vi "Autocomplete Demo.vi"() -> ()   [LabVIEW 2012]
doc: "This example includes a string XControl that probes the user input and checks it against a dynamic set of keywords. If what you type matches a keyword, the XControl autocompletes the word and selects the remaining portion of the word. This is also known as intellisense. At that point the you can tab to accept the autocompletion or keep typing to overwrite the completed portion.\n\nTo view the example:\n1) Run the VI.\n2) Type words in the <b>Intellisense Xcontrol</b> text box.\n\nYou can turn the Autocomplete function on or off as well as add new keywords to the Xcontrol."
uses:
  xcontrol/Intellisense Xcontrol.xctl
  xcontrol/Properties/Delimiter/Delimiter Enum.ctl
panel:
  in  "Keyword Dialog":bool
  in  "Delimiter":T1=enum."Space"
  in  "On/Off":bool=TRUE
  in  "Keyword Array":string[](array[string])
  in  "stop":bool
  out "Output Value":string
  in  "Intellisense Xcontrol":string(xcontrol)
  # "Select Help»Show Context Help and move the cursor \nover the VI icon to display help for this VI."
  # "Type text into the string control. If autocomplete is on and the text matches\na keyword, then the Xcontrol will autocomplete the keyword. To accept the\nautocompletion and add a delimiter, press tab. Otherwise, keep tying."
  # "Turn Autocomplete\non or off"
  # "Change the delimiter that\nseparates keywords"
  # "Add new keywords or\nchange the existing ones\nthat the Xcontrol searches\nfor by entering them into\nthe array of keywords."
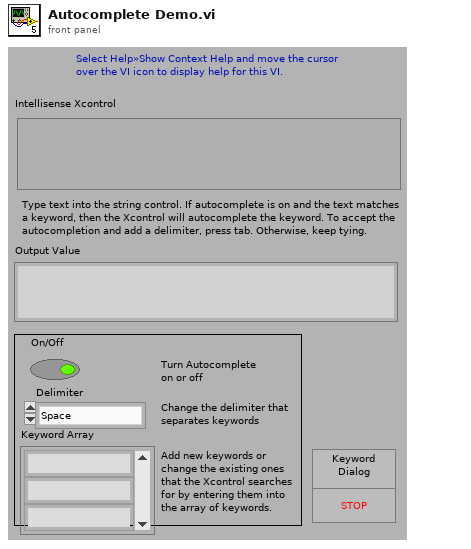
[diagram p1: front panel]
types:
  T1 = typedef "Intellisense Xcontrol.xctl/Delimiter Enum.ctl" = enum16{"None", "Space", "Dash \"-\"", "Slash \"/\"", "Backslash \"\\\"", "Colon", "Period", "Comma", "Line Feed"}
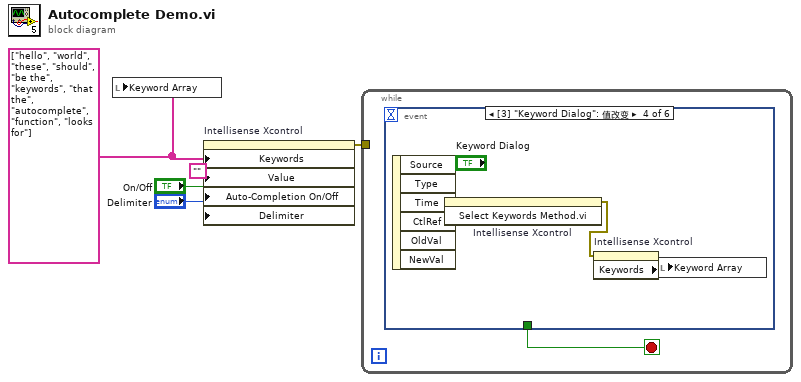
[diagram p0: block diagram]
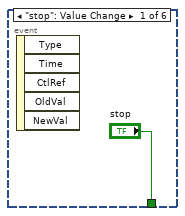
[diagram p2: hidden frame]
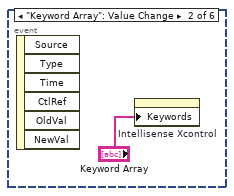
[diagram p3: hidden frame]
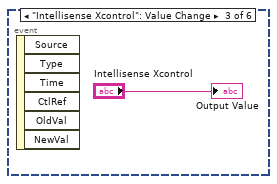
[diagram p4: hidden frame]
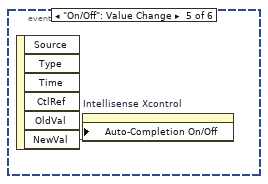
[diagram p5: hidden frame]
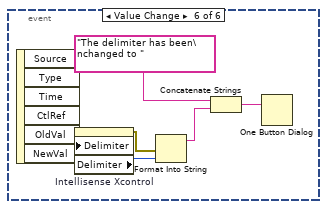
[diagram p6: hidden frame]
diagram:
  w2 = string[] ["hello", "world", "these", "should", "be the", "keywords", "that the", "autocomplete", "function", "looks for"] ("Keywords")
  n1 = local write "Keyword Array"(w2) -> ()
  n2 = property on="Intellisense Xcontrol" class="Intellisense Xcontrol (严格)"("Keywords"=w2, "Value"="", "Auto-Completion On/Off"="On/Off", "Delimiter"="Delimiter") -> (error out=w5:errorcluster)  [unwired: 2 in, 1 out]
  n3 = while {
    tunnel: w5 -> [_]
    stop <- w6 stop-if-true
    n4 = event shown="[3] \"Keyword Dialog\": 值改变" {
      selector: _ -> [_ _ _ _ _ _]
      dyn-events: _ -> [_ _ _ _ _ _]
      timeout: _ -> [_ _ _ _ _ _]
      tunnel: ["stop" _ _ _ _ _] -> w6
      event "stop": Value Change {
        n5 = event-data() -> ()  [unwired: 1 in, 5 out]
      }
      event "Keyword Array": Value Change {
        n6 = event-data() -> ()  [unwired: 1 in, 6 out]
        n7 = property on="Intellisense Xcontrol" class="Intellisense Xcontrol (严格)"("Keywords"="Keyword Array") -> ()  [unwired: 2 in, 2 out]
      }
      event "Intellisense Xcontrol": Value Change {
        n8 = event-data() -> ()  [unwired: 1 in, 6 out]
        "Output Value" <- "Intellisense Xcontrol"
      }
      event "Keyword Dialog": Value Change {
        n9 = event-data() -> ()  [unwired: 1 in, 6 out]
        n10 = invoke on="Intellisense Xcontrol" class="Intellisense Xcontrol (strict)" method="Select Keywords Method.vi"() -> (error out=w11:errorcluster)  [unwired: 3 in, 2 out]
        n11 = property on="Intellisense Xcontrol" class="Intellisense Xcontrol (严格)"(error in=w11) -> ("Keywords"=w10:string[])  [unwired: 1 in, 2 out]
        n12 = local write "Keyword Array"(w10) -> ()
      }
      event "On/Off": Value Change {
        n13 = event-data() -> ("NewVal"=w12:bool)  [unwired: 1 in, 5 out]
        n14 = property on="Intellisense Xcontrol" class="Intellisense Xcontrol (严格)"("Auto-Completion On/Off"=w12) -> ()  [unwired: 2 in, 2 out]
      }
      event Value Change {
        n15 = event-data() -> ("NewVal"=w18:T1)  [unwired: 1 in, 5 out]
        n16 = property on="Intellisense Xcontrol" class="Intellisense Xcontrol (严格)"("Delimiter"=w18) -> (error out=w17:errorcluster, "Delimiter"=w16:T1)  [unwired: 2 in, 1 out]
        n17 = Format Into String(error in=w17, w16) -> (resulting string=w14:string)  [unwired: 2 in, 1 out]
        n18 = Concatenate Strings("The delimiter has been\nchanged to " ("String"), w14) -> (w13:string)
        n19 = One Button Dialog(message=w13) -> ()  [unwired: 1 in, 1 out]
      }
    }
  }
